vi "SHA_calc_appendsU64.vi"(11 "String length":i32) -> (2 "Append":u8[](array[numeric]), 3 "Number of chunks":i32)   [LabVIEW 2011, in "i3-external-encryption.lvlib"]
doc: "Calculates the appendices for the last chunks (64-bit).\n\n(c) Ton Plomp, 2011\nTHIS SOFTWARE IS PROVIDED AS IS, AND ANY WARRANTY IS REJECTED"
uses:
  i3-external-encryption.lvlib
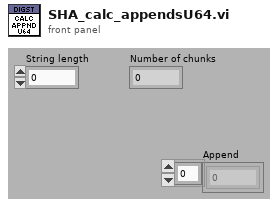
[diagram p1: front panel]
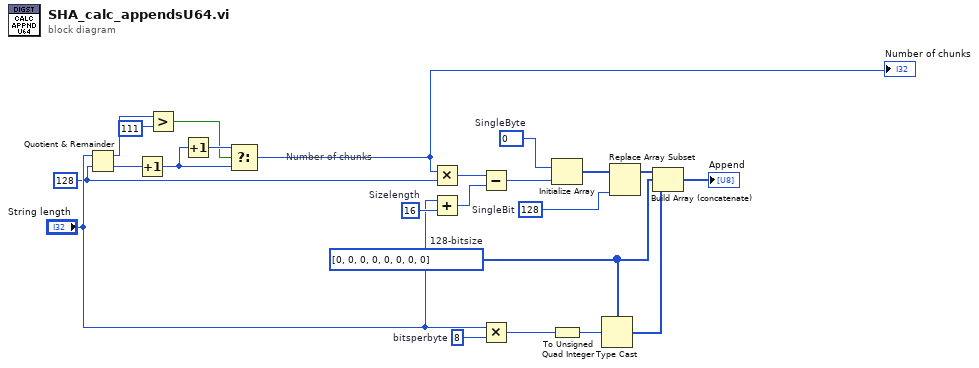
[diagram p0: block diagram]
diagram:
  w3 = u8[] [0, 0, 0, 0, 0, 0, 0, 0]  # 128-bitsize
  w6 = u8 0  # SingleByte
  w7 = u8 128  # SingleBit
  w15 = 16  # Sizelength
  w8 = 8  # bitsperbyte
  w12 = 128 ("y")
  # "Number of chunks"
  n1 = Quotient & Remainder(x="String length", y=w12) -> (x-y*floor(x/y)=w20:i32, floor(x/y)=w17:i32)
  n2 = Increment(x=w17) -> (x+1=w22:i32)
  n3 = Greater?(x=w20, y=111) -> (0:w1:bool)
  n4 = Increment(x=w22) -> (x+1=w21:i32)
  n5 = Select(t=w21, s=w1, f=w22) -> (s? t:f=w23:i32)
  "Number of chunks" <- w23
  n6 = Multiply(x=w23, y=w12) -> (x*y=w18:i32)
  n7 = Add(x="String length", y=w15) -> (x+y=w13:i32)
  n8 = Subtract(x=w18, y=w13) -> (x-y=w16:i32)
  n9 = Multiply(x="String length", y=w8) -> (x*y=w9:i32)
  n10 = Initialize Array(w6, w16) -> (w10:u8[])
  n11 = To Unsigned Quad Integer(1:w9) -> (0:w5:u64)
  n12 = Type Cast(type=w3, x=w5) -> (*(type *) &x=w4:u8[])
  n13 = Replace Array Subset(array=w10, new element=w7) -> (w11:u8[])  [unwired: 1 in]
  n14 = Build Array (concatenate)(w11, w3, w4) -> (→"Append":u8[])
